vi "Chimes.vi"(8 "error in":errorcluster) -> (0 "error out":errorcluster)   [LabVIEW 2020]
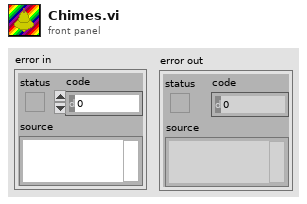
[diagram p1: front panel]
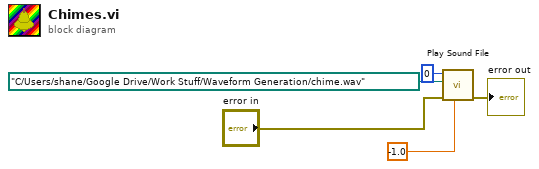
[diagram p0: block diagram]
diagram:
  n1 = call <vilib>:"Play Sound File.vi"("timeout (sec)"=-1.0, "error in (no error)"="error in", "path"=path "C:/Users/shane/Google Drive/Work Stuff/Waveform Generation/chime.wav", "device ID"=u32 0) -> ("error out"=→"error out":errorcluster)  [unwired: 6 in, 1 out]
